vi "unpack_eet.vi"(11 "payload":u64) -> (0 "lrv":sgl[](array[numeric]), 1 "right_ray":sgl[](array[numeric]), 2 "left_ray":sgl[](array[numeric]), 3 "combined_ray":sgl[](array[numeric]), 4 "error":bool, 5 "valid":u32)   [LabVIEW 2023]
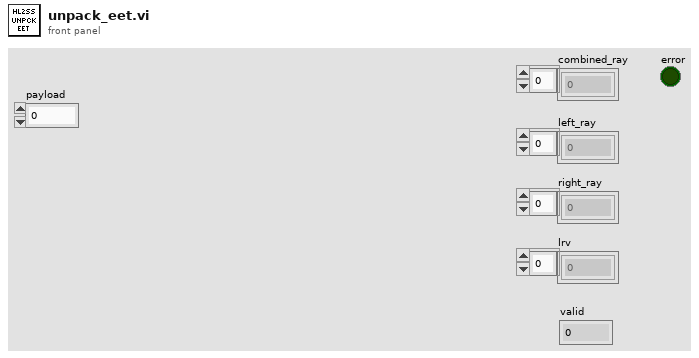
[diagram p1: front panel]
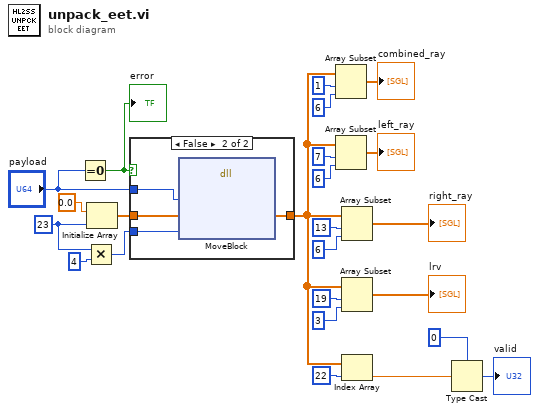
[diagram p0: block diagram]
diagram:
  w21 = 23 ("dimension size")
  n1 = Equal To 0?(x="payload") -> (x = 0?=w24:bool)
  "error" <- w24
  n2 = Multiply(x=w21, y=4) -> (x*y=w19:i32)
  n3 = Initialize Array(sgl 0.0 ("element"), w21) -> (w22:sgl[])
  n4 = case shown="False" w24 {
    tunnel: "payload" -> [_ w27]
    tunnel: w22 -> [w25 w29]
    tunnel: w19 -> [_ w28]
    tunnel: [w25 w26] -> w4
    frame True {
    }
    frame False {
      n5 = dll-call lib="LabVIEW" fn="MoveBlock"("ps"=w27, "pd"=w29, "size"=w28) -> ("pd"=w26:sgl[])  [unwired: 6 in, 2 out]
    }
  }
  n6 = Array Subset(array=w4, index=1, length=6) -> (→"combined_ray":sgl[])
  n7 = Array Subset(array=w4, index=7, length=6) -> (→"left_ray":sgl[])
  n8 = Array Subset(array=w4, index=13, length=6) -> (→"right_ray":sgl[])
  n9 = Array Subset(array=w4, index=19, length=3) -> (→"lrv":sgl[])
  n10 = Index Array(array=w4, index=22) -> (element=w9:sgl)
  n11 = Type Cast(type=u32 0 ("index"), x=w9) -> (*(type *) &x=→"valid":u32)
